vi "Generate Command Object.vi"(3 "data in":string) -> (1 "Remote Access Commands.lvclass":refnum<class "Remote Access Commands.lvclass">)   [LabVIEW 2015, in "Startup Processes.lvlib" / "Remote Access Commands.lvclass"]
uses:
  Remote Access Commands.lvclass
  _typedefs/Set Acquisiton Rate Input Cluster.ctl
  Set Acquisition Rate/Remote Access Commands_Set Acquisition Rate.lvclass
  _typedefs/Set Data Buffer Depth Input Cluster.ctl
  Set Data Buffer Depth/Remote Access Commands_Set Data Buffer Depth.lvclass
  _typedefs/Set TC Parameters Input Cluster.ctl
  _typedefs/TC Setup Parameters.ctl
  Set TC Parameters/Remote Access Commands_Set TC Parameters.lvclass
  _typedefs/Get Graph Data Input Cluster.ctl
  Read Graph Data/Remote Access Commands_Read Graph Data.lvclass
  _typedefs/Get Graph Image Input Cluster.ctl
  Read Graph Image/Remote Access Commands_Read Graph Image.lvclass
  Startup Processes.lvlib
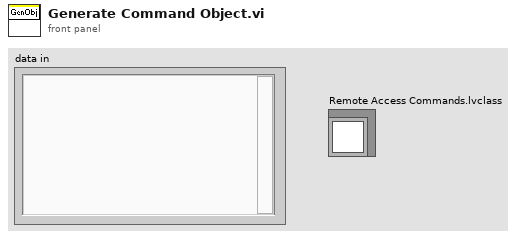
[diagram p1: front panel]
types:
  T1 = typedef "Startup Processes.lvlib/Remote Access Commands.lvclass/Set Acquisiton Rate Input Cluster.ctl" = cluster{"Target":string, "Interval":i32}
  T2 = typedef "Startup Processes.lvlib/Remote Access Commands.lvclass/Set Data Buffer Depth Input Cluster.ctl" = cluster{"Target":string, "Depth":i32}
  T3 = typedef "Startup Processes.lvlib/Remote Access Commands.lvclass/Set TC Parameters Input Cluster.ctl" = cluster{"Target":string, "Params":T4}
  T4 = typedef "Startup Processes.lvlib/TC Setup Parameters.ctl" = cluster{"Error High Level":dbl, "Warning High Level":dbl, "Warning Low Level":dbl, "Error Low Level":dbl, "Sample Interval":dbl[unit]}
  T5 = typedef "Startup Processes.lvlib/Remote Access Commands.lvclass/Get Graph Data Input Cluster.ctl" = cluster{"Target":string}
  T6 = typedef "Startup Processes.lvlib/Remote Access Commands.lvclass/Get Graph Image Input Cluster.ctl" = cluster{"Target":string}
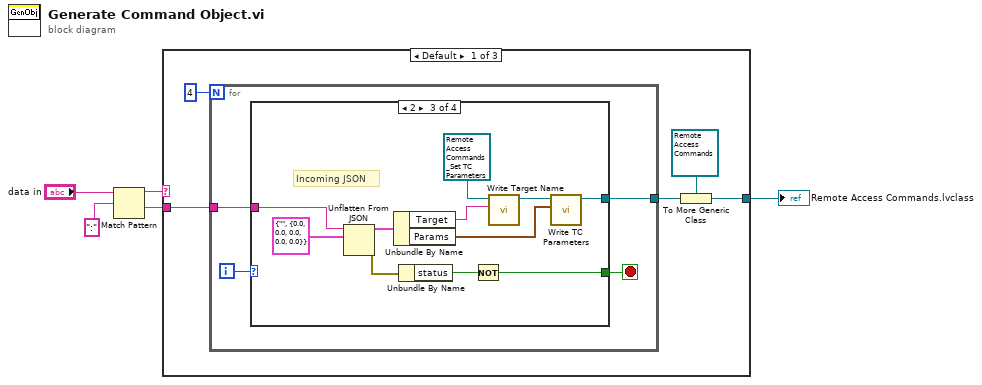
[diagram p0: block diagram]
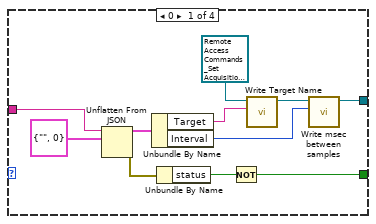
[diagram p2: hidden frame]
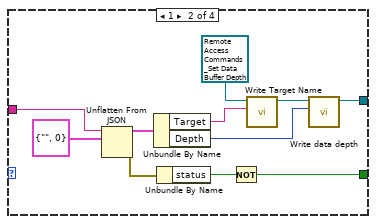
[diagram p3: hidden frame]
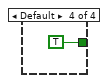
[diagram p4: hidden frame]
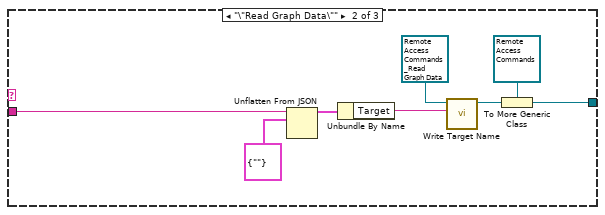
[diagram p5: hidden frame]
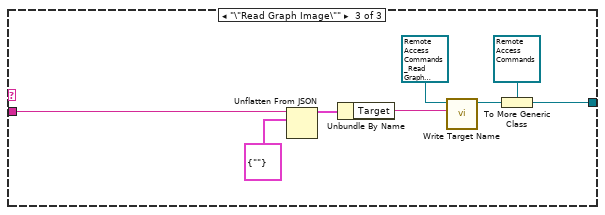
[diagram p6: hidden frame]
diagram:
  n1 = Match Pattern(string="data in", regular expression=":") -> (before substring=w4:string, after substring=w1:string)  [unwired: 1 in, 2 out]
  n2 = case shown="Default" w4 {
    tunnel: w1 -> [w6 w56 w64]
    tunnel: [w9 w50 w58] -> w3
    frame Default {
      n3 = for {
        N: 4 -> [_]
        tunnel: [w14] -> w8
        tunnel: w6 -> [w11]
        i -> [w13]
        stop <- w12 stop-if-true
        n4 = case shown="2" w13 {
          tunnel: [w16 w27 w37 _] -> w14
          tunnel: [w20 w31 w42 TRUE] -> w12
          tunnel: w11 -> [w24 w35 w46 _]
          frame 0 {
            n5 = Unflatten From JSON(JSON string=w24, type and defaults=T1 {"Target"="", "Interval"=0} ("Get Graph Data Input")) -> (value=w25:T1, error out=w22:errorcluster)  [unwired: 5 in]
            n6 = Unbundle By Name(w25) -> ("Target"=w19:string, "Interval"=w15:i32)
            n7 = Unbundle By Name(w22) -> ("status"=w21:bool)
            n8 = Not(x=w21) -> (.not. x?=w20:bool)
            n9 = call "Write Target Name.vi"("Target Name"=w19, "Remote Access Commands in"=refnum<class "Remote Access Commands_Set Acquisition Rate.lvclass"> refnum) -> ("Remote Access Commands out"=w17:refnum<class "Remote Access Commands_Set Acquisition Rate.lvclass">)  [unwired: 4 in, 1 out]
            n10 = call-dynamic "Write msec between samples.vi"("msec between samples"=w15, "Set Acquisition Rate in"=w17) -> ("Set Acquisition Rate out"=w16:refnum<class "Remote Access Commands_Set Acquisition Rate.lvclass">)  [unwired: 4 in, 1 out]
          }
          frame 1 {
            n11 = Unflatten From JSON(JSON string=w35, type and defaults=T2 {"Target"="", "Depth"=0} ("Get Graph Data Input")) -> (value=w36:T2, error out=w33:errorcluster)  [unwired: 5 in]
            n12 = Unbundle By Name(w36) -> ("Target"=w30:string, "Depth"=w26:i32)
            n13 = Unbundle By Name(w33) -> ("status"=w32:bool)
            n14 = Not(x=w32) -> (.not. x?=w31:bool)
            n15 = call "Write Target Name.vi"("Target Name"=w30, "Remote Access Commands in"=refnum<class "Remote Access Commands_Set Data Buffer Depth.lvclass"> refnum) -> ("Remote Access Commands out"=w28:refnum<class "Remote Access Commands_Set Data Buffer Depth.lvclass">)  [unwired: 4 in, 1 out]
            n16 = call-dynamic "Write data depth.vi"("data depth"=w26, "Set Data Buffer Depth in"=w28) -> ("Set Data Buffer Depth out"=w27:refnum<class "Remote Access Commands_Set Data Buffer Depth.lvclass">)  [unwired: 4 in, 1 out]
          }
          frame 2 {
            # "Incoming JSON"
            n17 = Unflatten From JSON(JSON string=w46, type and defaults=T3 {"Target"="", "Params"={"Error High Level"=0.0, "Warning High Level"=0.0, "Warning Low Level"=0.0, "Error Low Level"=0.0, "Sample Interval"=0.0}} ("Get Graph Data Input")) -> (value=w47:T3, error out=w44:errorcluster)  [unwired: 5 in]
            n18 = Unbundle By Name(w47) -> ("Target"=w41:string, "Params"=w38:T4)
            n19 = Unbundle By Name(w44) -> ("status"=w43:bool)
            n20 = Not(x=w43) -> (.not. x?=w42:bool)
            n21 = call "Write Target Name.vi"("Target Name"=w41, "Remote Access Commands in"=refnum<class "Remote Access Commands_Set TC Parameters.lvclass"> refnum) -> ("Remote Access Commands out"=w39:refnum<class "Remote Access Commands_Set TC Parameters.lvclass">)  [unwired: 4 in, 1 out]
            n22 = call-dynamic "Write TC Parameters.vi"("TC Parameters"=w38, "Set TC Parameters in"=w39) -> ("Set TC Parameters out"=w37:refnum<class "Remote Access Commands_Set TC Parameters.lvclass">)  [unwired: 4 in, 1 out]
          }
          frame Default {
          }
        }
      }
      n23 = To More Generic Class(target class=refnum<class "Remote Access Commands.lvclass"> refnum, reference=w8) -> (generic class reference=w9:refnum<class "Remote Access Commands.lvclass">)
    }
    frame "\"Read Graph Data\"" {
      n24 = Unflatten From JSON(JSON string=w56, type and defaults=T5 {"Target"=""} ("Get Graph Data Input")) -> (value=w54:T5)  [unwired: 5 in, 1 out]
      n25 = Unbundle By Name(w54) -> ("Target"=w52:string)
      n26 = call "Write Target Name.vi"("Target Name"=w52, "Remote Access Commands in"=refnum<class "Remote Access Commands_Read Graph Data.lvclass"> refnum) -> ("Remote Access Commands out"=w51:refnum<class "Remote Access Commands_Read Graph Data.lvclass">)  [unwired: 4 in, 1 out]
      n27 = To More Generic Class(target class=refnum<class "Remote Access Commands.lvclass"> refnum, reference=w51) -> (generic class reference=w50:refnum<class "Remote Access Commands.lvclass">)
    }
    frame "\"Read Graph Image\"" {
      n28 = Unflatten From JSON(JSON string=w64, type and defaults=T6 {"Target"=""} ("Get Graph Data Input")) -> (value=w62:T6)  [unwired: 5 in, 1 out]
      n29 = Unbundle By Name(w62) -> ("Target"=w60:string)
      n30 = call "Write Target Name.vi"("Target Name"=w60, "Remote Access Commands in"=refnum<class "Remote Access Commands_Read Graph Image.lvclass"> refnum) -> ("Remote Access Commands out"=w59:refnum<class "Remote Access Commands_Read Graph Image.lvclass">)  [unwired: 4 in, 1 out]
      n31 = To More Generic Class(target class=refnum<class "Remote Access Commands.lvclass"> refnum, reference=w59) -> (generic class reference=w58:refnum<class "Remote Access Commands.lvclass">)
    }
  }
  "Remote Access Commands.lvclass" <- w3
